vi "DSF.Engine.Framework.Set Runtime.vi"(8 "error in (no error)":errorcluster, 10 "Framework Runtime":refnum<class "DSF.Engine.Runtime.Framework.lvclass">, 11 "Framework in":refnum<class "Framework.lvclass">) -> (0 "error out":errorcluster, 3 "Framework out":refnum<class "Framework.lvclass">)   [LabVIEW 2016, in "DSF.Engine.lvlib" / "Framework.lvclass"]
uses:
  Framework.lvclass
  DSF.Engine.Runtime.Framework.lvclass
  Framework.lvclass/Framework.ctl
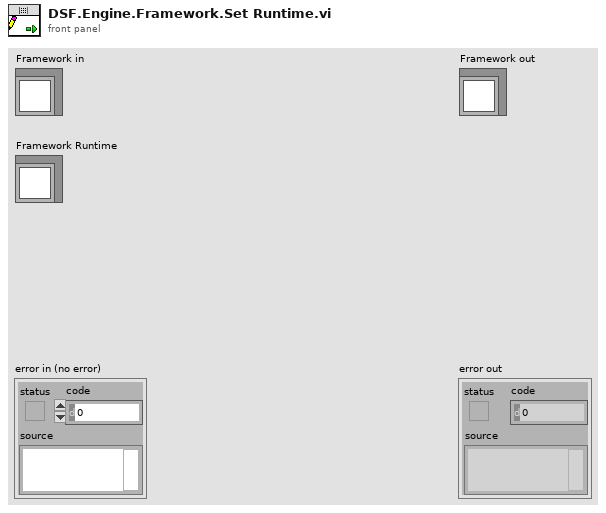
[diagram p1: front panel]
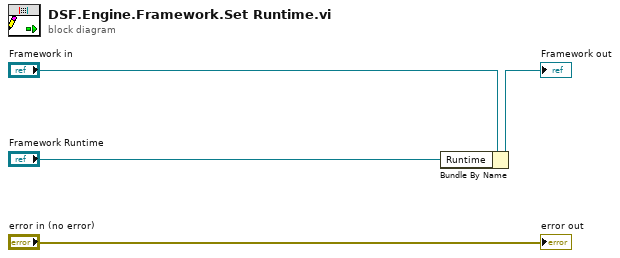
[diagram p0: block diagram]
diagram:
  n1 = Bundle By Name(cluster="Framework in", "Runtime"="Framework Runtime") -> (→"Framework out":refnum<class "Framework.lvclass">)
  "error out" <- "error in (no error)"
